vi "Execute.vi"(8 "error in (no error)":errorcluster, 10 "System In":refnum<class "abs_System.lvclass">, 11 "Node in":refnum<class "Repeater.lvclass">) -> (0 "error out":errorcluster, 1 "Status":T1, 2 "System Out":refnum<class "abs_System.lvclass">, 3 "Node out":refnum<class "Repeater.lvclass">)   [LabVIEW 2021, in "BT.lvlib" / "Repeater.lvclass"]
uses:
  Repeater.lvclass
  abs_Node/Status.ctl
  abs_System/abs_System.lvclass
  Repeater.lvclass/Repeater.ctl
  abs_Decorator/abs_Decorator.lvclass
  abs_Node/abs_Node.lvclass
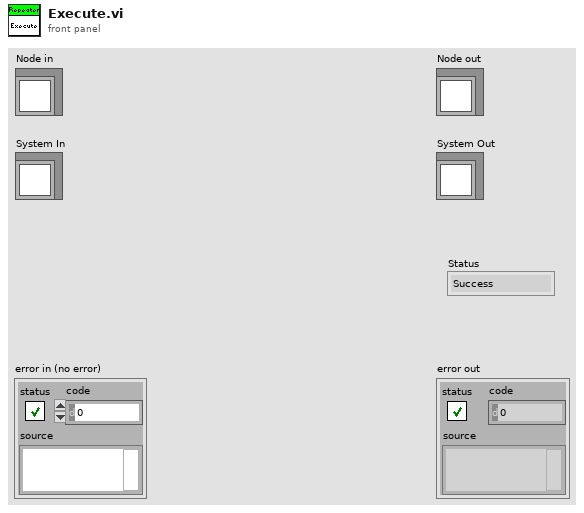
[diagram p1: front panel]
types:
  T1 = typedef "BT.lvlib/abs_Node.lvclass/Status.ctl" = enum16{"Success", "Failure", "Running"}
  T2 = typedef "BT.lvlib/Repeater.lvclass/Finish On - Type.ctl" = enum16{"Success", "Failure", "Never"}
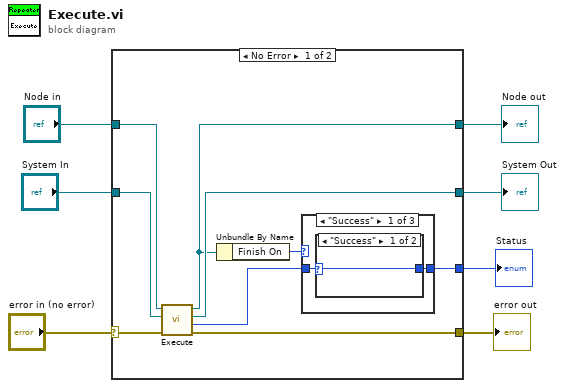
[diagram p0: block diagram]
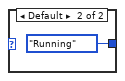
[diagram p2: hidden frame]
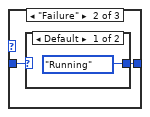
[diagram p3: hidden frame]
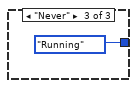
[diagram p5: hidden frame]
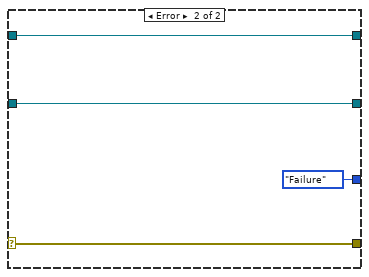
[diagram p6: hidden frame]
diagram:
  n1 = case shown="No Error" "error in (no error)" {
    selector: "error in (no error)" -> [w15 w29]
    tunnel: [w16 w28] -> w7
    tunnel: "System In" -> [w14 w28]
    tunnel: "Node in" -> [w13 w27]
    tunnel: [w12 w27] -> w3
    tunnel: [w9 Status."Failure" ("Status")] -> w2
    tunnel: [w8 w29] -> w1
    frame No Error {
      n2 = call-parent "Execute.vi"("error in (no error)"=w15, "System In"=w14, "Node in"=w13) -> ("error out"=w8:errorcluster, "Status"=w10:T1, "System Out"=w16:refnum<class "abs_System.lvclass">, "Node out"=w12:refnum<class "Repeater.lvclass">)  [unwired: 5 in]
      n3 = Unbundle By Name(w12) -> ("Finish On"=w11:T2)
      n4 = case shown="\"Success\"" w11 {
        tunnel: w10 -> [w17 w21 _]
        tunnel: [w18 w22 Status."Running" ("Status")] -> w9
        frame "Success" {
          n5 = case shown="\"Success\"" w17 {
            selector: w17 -> [w19 _]
            tunnel: [w19 Status."Running" ("Status")] -> w18
            frame "Success" {
            }
            frame Default {
            }
          }
        }
        frame "Failure" {
          n6 = case shown="Default" w21 {
            selector: w21 -> [_ w24]
            tunnel: [Status."Running" ("Status") w24] -> w22
            frame Default {
            }
            frame "Failure" {
            }
          }
        }
        frame "Never" {
        }
      }
    }
    frame Error {
    }
  }
  "error out" <- w1
  "Node out" <- w3
  "Status" <- w2
  "System Out" <- w7
